vi "spDevice_readData.vi"(5 "Dont wait":bool, 7 "Number of records":u32, 8 "error in (no error)":errorcluster, 9 "Trigger":enum32{"Software", "Level", "External"}(radio), 10 "Samples per record":u32, 11 "adq_cu_ptr in":u32) -> (0 "error out":errorcluster, 2 "Done reading":bool, 3 "adq_cu_ptr out":u32, 4 "buffer_chB_out":i16[](array[numeric]), 6 "buffer_chA_out":i16[](array[numeric]))   [LabVIEW 2013]
doc: "Acquires the 'number of samples per run' repeatedly using the chosen trigger. \nOutputs arrays of the memory buffers read from Channel A and Channel B. Remember to parse them into individual records"
uses:
  turn_off_global_variable.vi
panel:
  # "VI Output"
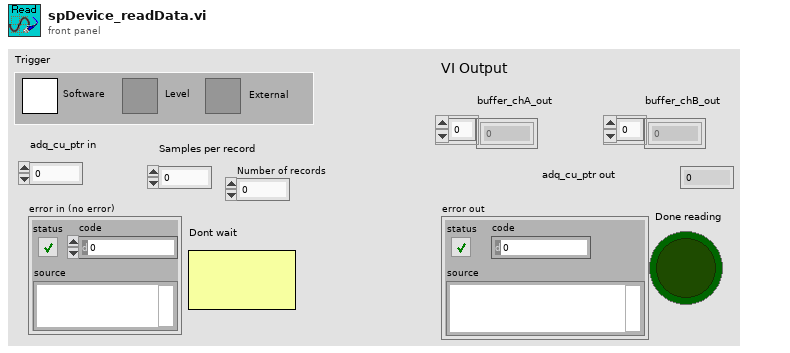
[diagram p1: front panel]
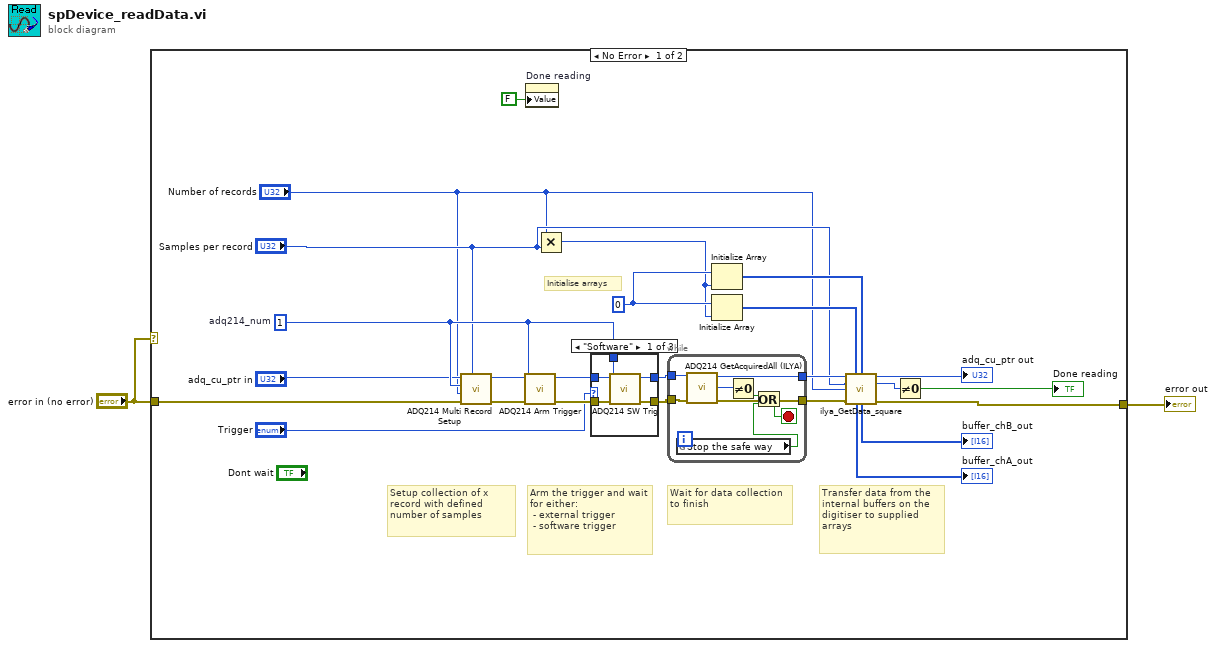
[diagram p0: block diagram]
diagram:
  n1 = case shown="No Error" "error in (no error)" {
    tunnel: "error in (no error)" -> [w18 w45]
    tunnel: [w3 w45] -> w1
    frame No Error {
      w23 = 1  # adq214_num
      w10 = i16 0 ("dimension size")
      # "Initialise arrays"
      # "Transfer data from the internal buffers on the digitiser to supplied arrays"
      # "Wait for data collection to finish"
      # "Arm the trigger and wait for either:\n - external trigger\n - software trigger"
      # "Setup collection of x record with defined number of samples"
      n2 = call "ADQ214 Multi Record Setup.vi"("SamplesPerRecord"="Samples per record", "error in (no error)"=w18, "NumberOfRecords"="Number of records", "adq214_num"=w23, "adq_cu_ptr"="adq_cu_ptr in") -> ("error out"=w25:errorcluster, "adq_cu_ptr out"=w24:u32)  [unwired: 4 in, 1 out]
      n3 = call "ADQ214 Arm Trigger.vi"("error in (no error)"=w25, "adq214_num"=w23, "adq_cu_ptr"=w24) -> ("error out"=w22:errorcluster, "adq_cu_ptr out"=w21:u32)  [unwired: 6 in, 1 out]
      n4 = property on="Done reading" class="Bool (strict)"("Value"=FALSE ("Done reading")) -> ()  [unwired: 2 in, 2 out]
      n5 = Multiply(x="Number of records", y="Samples per record") -> (x*y=w9:u32)
      n6 = case shown="\"Software\"" "Trigger" {
        tunnel: [w32 w33 w35] -> w27
        tunnel: [w31 w34 w36] -> w26
        tunnel: w23 -> [w30 _ _]
        tunnel: w22 -> [w29 w33 w35]
        tunnel: w21 -> [w28 w34 w36]
        frame "Software" {
          n7 = call "ADQ214 SW Trig.vi"("error in (no error)"=w29, "adq214_num"=w30, "adq_cu_ptr"=w28) -> ("error out"=w32:errorcluster, "adq_cu_ptr out"=w31:u32)  [unwired: 6 in, 1 out]
        }
        frame "Level" {
        }
        frame "External" {
        }
      }
      n8 = while {
        tunnel: w26 -> [w42]
        tunnel: w27 -> [w38]
        tunnel: [w41] -> w8
        tunnel: [w40] -> w15
        stop <- w43 stop-if-true
        n9 = global read "turn_off_global_variable.vi" "Stop the safe way"() -> (w37:bool)
        n10 = call "ADQ214 GetAcquiredAll (ILYA).vi"("error in"=w38, "adq_cu_ptr"=w42) -> ("error out"=w40:errorcluster, "return"=w39:u32, "adq_cu_ptr"=w41:u32)  [unwired: 7 in]
        n11 = Not Equal To 0?(x=w39) -> (x != 0?=w44:bool)
        n12 = Or(x=w44, y=w37) -> (x .or. y?=w43:bool)
      }
      n13 = Initialize Array(w10, w9) -> (w11:i16[])
      n14 = Initialize Array(w10, w9) -> (w12:i16[])
      n15 = call "ilya_GetData_square.vi"("adq_cu_ptr"=w8, "buffer_chA_in"=w12, "buffer_chB_in"=w11, "samples_per_record"="Samples per record", "number_of_records"="Number of records", "error in"=w15) -> ("adq_cu_ptr"=→"adq_cu_ptr out":u32, "function return"=w13:i32, "buffer_chA_out"=→"buffer_chA_out":i16[], "buffer_chB_out"=→"buffer_chB_out":i16[], "error out"=w3:errorcluster)  [unwired: 5 in]
      n16 = Not Equal To 0?(x=w13) -> (x != 0?=→"Done reading":bool)
    }
    frame Error {
    }
  }
  "error out" <- w1
